vi "CreateServiceFolder.vi"(2 "element":string, 3 "selected path":path) -> (0 "cancelled":bool, 1 "created path":path)   [LabVIEW 2019]
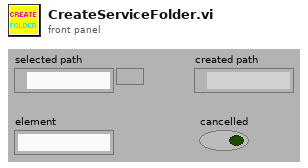
[diagram p1: front panel]
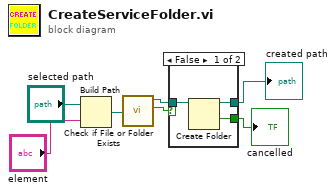
[diagram p0: block diagram]
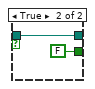
[diagram p2: hidden frame]
diagram:
  n1 = Build Path(base path="selected path", name or relative path="element") -> (appended path=w5:path)
  n2 = call <vilib>:"Check if File or Folder Exists.vi"("path"=w5) -> ("file or folder exists?"=w7:bool, "dup path"=w6:path)  [unwired: 8 in, 1 out]
  n3 = case shown="False" w7 {
    tunnel: [w10 w12] -> w1
    tunnel: [w9 FALSE ("cancelled")] -> w2
    tunnel: w6 -> [w8 w12]
    frame False {
      n4 = Create Folder(path (use dialog)=w8) -> (created path=w10:path, cancelled=w9:bool)  [unwired: 2 in, 1 out]
    }
    frame True {
    }
  }
  "cancelled" <- w2
  "created path" <- w1
